vi "Moving average.vi"(2 "Central mAV t/f (t)":bool=TRUE, 3 "Width of AV":i32=10, 4 "Raw data":dbl[](array[numeric])=[1.0]) -> (0 "Data STDEVs":dbl[](array[numeric]), 1 "Data AVs":dbl[](array[numeric]))   [LabVIEW 2010]
doc: "Written by Matthew Partridge 2011"
uses:
  <vilib>/Analysis/NI_AALBase.lvlib
panel:
  # "Takes a 1D array and applies a moving average\neither as a central point (taking account of n/2 points either side) or as a simple moving average (using the previous n points)"
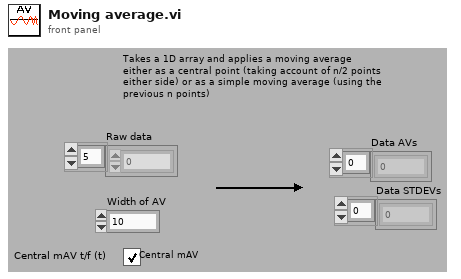
[diagram p1: front panel]
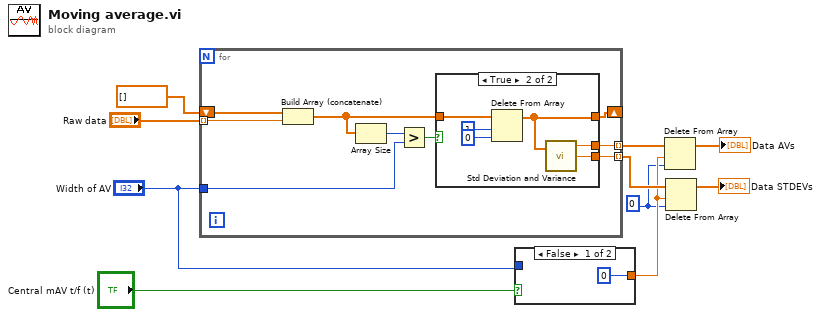
[diagram p0: block diagram]
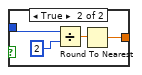
[diagram p2: hidden frame]
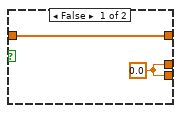
[diagram p3: hidden frame]
diagram:
  w5 = 0
  n1 = for {
    tunnel: "Raw data" -> [w11] mode=indexing
    shift-right: [w14] -> _
    shift-left: dbl[] [] -> [w19]
    tunnel: "Width of AV" -> [w18]
    tunnel: [w12] -> w8 mode=indexing
    tunnel: [w13] -> w9 mode=indexing
    n2 = Build Array (concatenate)(w19, w11) -> (w15:dbl[])
    n3 = Array Size(array=w15) -> (size(s)=w17:i32)
    n4 = Greater?(x=w17, y=w18) -> (0:w16:bool)
    n5 = case shown="True" w16 {
      tunnel: w15 -> [w21 w27]
      tunnel: [w21 w22] -> w14
      tunnel: [w20 w24] -> w13
      tunnel: [w20 w23] -> w12
      frame False {
        w20 = sgl 0.0
      }
      frame True {
        n6 = Delete From Array(array=w27, length=1, index=0) -> (array with subset deleted=w22:dbl[])  [unwired: 1 out]
        n7 = call <vilib>:"Std Deviation and Variance.vi"("X"=w22) -> ("mean"=w24:dbl, "standard deviation"=w23:dbl)  [unwired: 1 in, 1 out]
      }
    }
  }
  n8 = case shown="False" "Central mAV t/f (t)" {
    tunnel: "Width of AV" -> [_ w30]
    tunnel: [0 w29] -> w6
    frame False {
    }
    frame True {
      n9 = Divide(x=w30, y=2) -> (x/y=w31:dbl)
      n10 = Round To Nearest(number=w31) -> (nearest integer value=w29:dbl)
    }
  }
  n11 = Delete From Array(array=w9, length=w6, index=w5) -> (array with subset deleted=→"Data AVs":dbl[])  [unwired: 1 out]
  n12 = Delete From Array(array=w8, length=w6, index=w5) -> (array with subset deleted=→"Data STDEVs":dbl[])  [unwired: 1 out]
